vi "Parametric Viewer.vi"(8 "Error In":errorcluster, 11 "F6XX_In":T1) -> (0 "Error Out":errorcluster, 3 "F6XX_Out":T1)   [LabVIEW 2023]
uses:
  type defs/F6_ERD_Control.ctl
panel:
  in  "?":enum32{"F6XX"}(tab)
  in  "Stop":bool
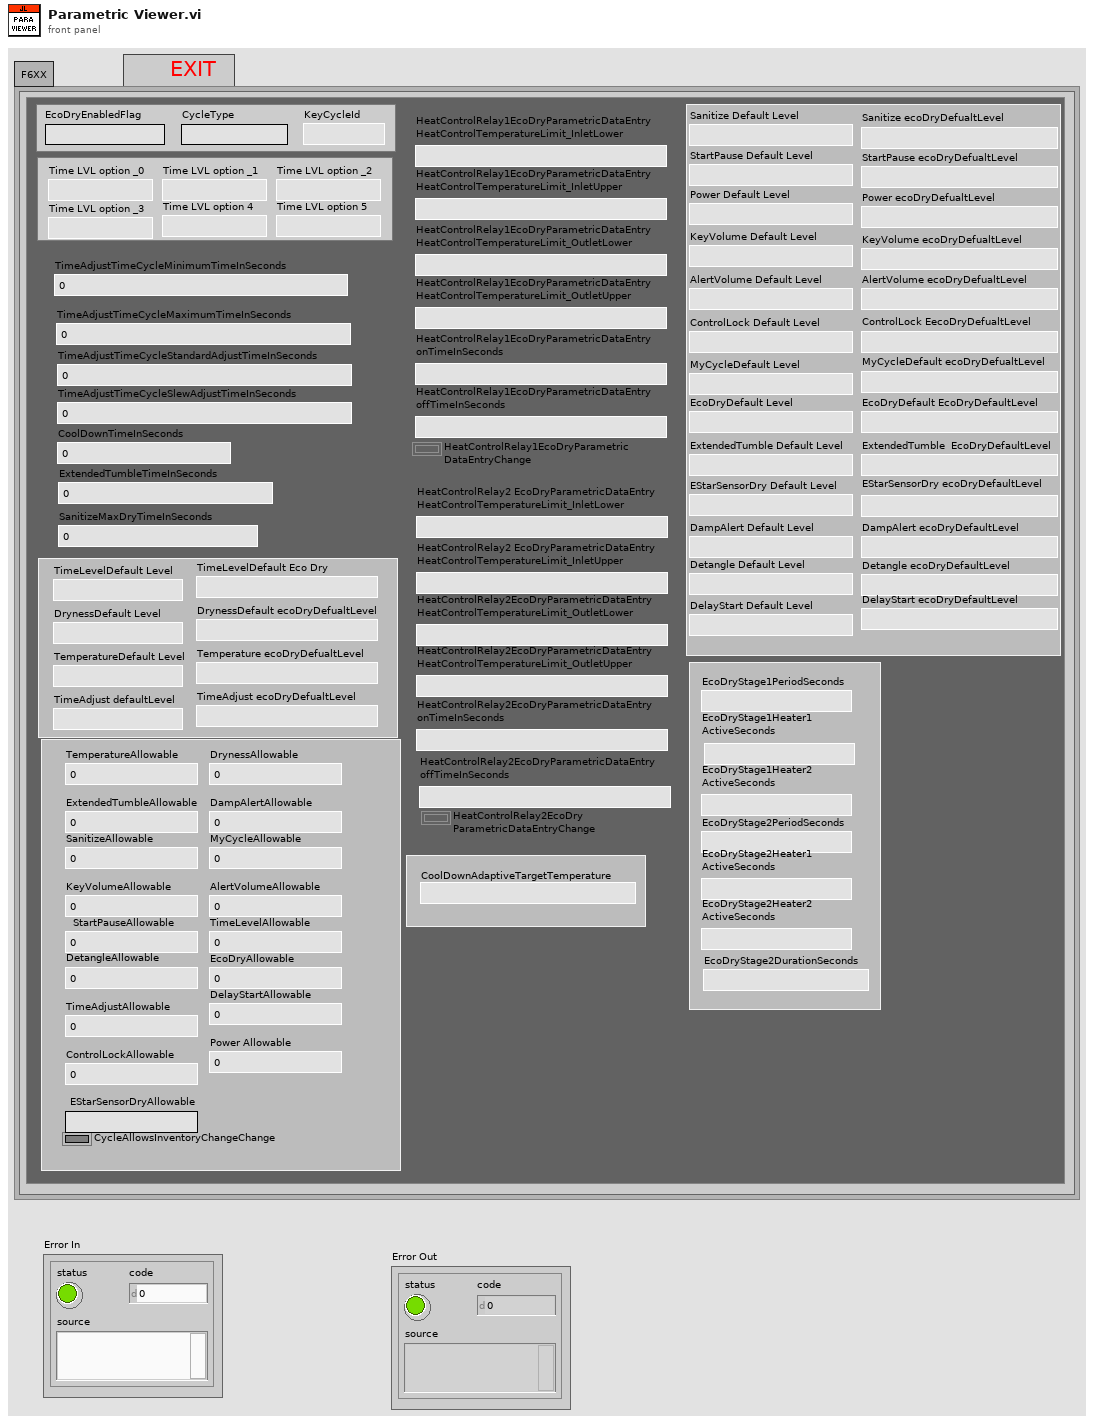
[diagram p1: front panel]
types:
  T1 = typedef "F6_ERD_Control.ctl" = cluster{"EcoDryEnabledFlag":string, "KeyCycleId":u8, "CycleType":string, "Time LVL option 5":u32, "Time LVL option 4":u32, "Time LVL option _3":u32, "Time LVL option _2":u32, "Time LVL option _1":u32, "Time LVL option _0":u32, "CoolDownTimeInSeconds":u32, "TimeAdjustTimeCycleMinimumTimeInSeconds":u32, "TimeAdjustTimeCycleMaximumTimeInSeconds":u32, "TimeAdjustTimeCycleStandardAdjustTimeInSeconds":u32, "TimeAdjustTimeCycleSlewAdjustTimeInSeconds":u32, "ExtendedTumbleTimeInSeconds":u32, "SanitizeMaxDryTimeInSeconds":u32, "TemperatureDefault Level":u8, "Temperature ecoDryDefualtLevel":u8, "DrynessDefault Level":u8, "DrynessDefault ecoDryDefualtLevel":u8, "TimeAdjust defaultLevel":u8, "TimeAdjust ecoDryDefualtLevel":u8, "TimeLevelDefault Level":u8, "TimeLevelDefault Eco Dry":u8, "EStarSensorDry Default Level":u8, "EStarSensorDry ecoDryDefaultLevel":u8, "EcoDryDefault Level":u8, "EcoDryDefault EcoDryDefaultLevel ":u8, "ExtendedTumble Default Level":u8, "ExtendedTumble  EcoDryDefaultLevel":u8, "Sanitize Default Level":u8, "Sanitize ecoDryDefualtLevel":u8, "MyCycleDefault Level":u8, "MyCycleDefault ecoDryDefualtLevel":u8, "StartPause Default Level":u8, "StartPause ecoDryDefualtLevel":u8, "Power Default Level":u8, "Power ecoDryDefualtLevel":u8, "KeyVolume Default Level":u8, "KeyVolume ecoDryDefualtLevel":u8, "AlertVolume Default Level":u8, "AlertVolume ecoDryDefualtLevel":u8, "ControlLock Default Level":u8, "ControlLock EecoDryDefualtLevel":u8, "HeatControlRelay1EcoDryParametricDataEntry\nHeatControlTemperatureLimit_InletLower":u16, "HeatControlRelay1EcoDryParametricDataEntry\nHeatControlTemperatureLimit_InletUpper":u16, "HeatControlRelay1EcoDryParametricDataEntry\nHeatControlTemperatureLimit_OutletLower":u16, "HeatControlRelay1EcoDryParametricDataEntry\nHeatControlTemperatureLimit_OutletUpper":u16, "HeatControlRelay1EcoDryParametricDataEntry\nonTimeInSeconds":u8, "HeatControlRelay1EcoDryParametricDataEntry\noffTimeInSeconds":u8, "HeatControlRelay1EcoDryParametric\nDataEntryChange ":bool, "HeatControlRelay2 EcoDryParametricDataEntry\nHeatControlTemperatureLimit_InletLower":u16, "HeatControlRelay2 EcoDryParametricDataEntry\nHeatControlTemperatureLimit_InletUpper ":u16, "HeatControlRelay2EcoDryParametricDataEntry\nHeatControlTemperatureLimit_OutletLower ":u16, "HeatControlRelay2EcoDryParametricDataEntry\nHeatControlTemperatureLimit_OutletUpper":u16, "HeatControlRelay2EcoDryParametricDataEntry\nonTimeInSeconds ":u8, "HeatControlRelay2EcoDryParametricDataEntry\noffTimeInSeconds ":u8, "HeatControlRelay2EcoDry\nParametricDataEntryChange":bool, "DampAlert Default Level":u8, "DampAlert ecoDryDefaultLevel":u8, "Detangle Default Level ":u8, "Detangle ecoDryDefaultLevel":u8, "DelayStart Default Level":u8, "DelayStart ecoDryDefaultLevel":u8, "CycleAllowsInventoryChangeChange":bool, "TemperatureAllowable":u8, "DrynessAllowable":u8, "TimeLevelAllowable":u8, "EcoDryAllowable":u8, "ExtendedTumbleAllowable":u8, "DampAlertAllowable":u8, "DetangleAllowable":u8, "DelayStartAllowable":u8, "SanitizeAllowable":u8, "MyCycleAllowable":u8, "TimeAdjustAllowable":u8, "Power Allowable":u8, "KeyVolumeAllowable":u8, "AlertVolumeAllowable":u8, "ControlLockAllowable":u8, "EStarSensorDryAllowable":string, "StartPauseAllowable":u8, "EcoDryStage1Heater2\nActiveSeconds":u32, "EcoDryStage2PeriodSeconds":u32, "EcoDryStage2Heater1\nActiveSeconds":u32, "EcoDryStage2Heater2\nActiveSeconds":u32, "EcoDryStage1Heater1\nActiveSeconds":u32, "EcoDryStage1PeriodSeconds":u32, "EcoDryStage2DurationSeconds":u32, "CoolDownAdaptiveTargetTemperature":u16}
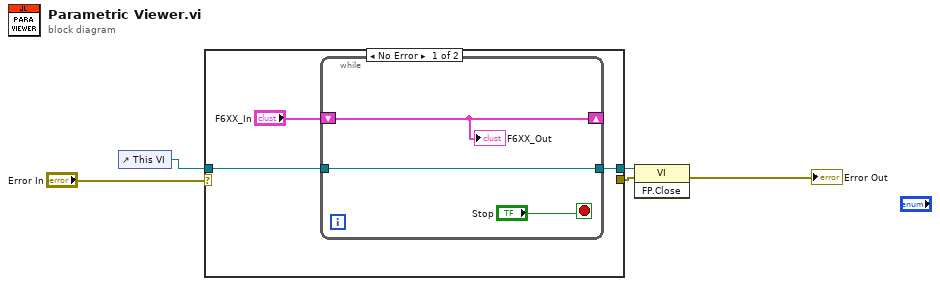
[diagram p0: block diagram]
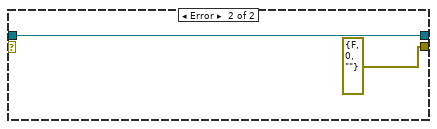
[diagram p2: hidden frame]
diagram:
  n1 = control-ref of="This VI"() -> (w4:refnum<vi>)
  n2 = case shown="No Error" "Error In" {
    tunnel: [w8 w13] -> w5
    tunnel: w4 -> [w6 w13]
    tunnel: [_ errorcluster {"status"=FALSE, "code"=0, "source"=""} ("error IO")] -> w1
    frame No Error {
      n3 = while {
        tunnel: [w9] -> w8
        shift-right: [w10] -> _
        shift-left: "F6XX_In" -> [w10]
        tunnel: w6 -> [w9]
        stop <- "Stop" stop-if-true
        "F6XX_Out" <- w10
      }
    }
    frame Error {
    }
  }
  n4 = invoke class="VI" method="FP.Close"(reference=w5, error in=w1) -> (error out=→"Error Out":errorcluster)  [unwired: 1 in, 2 out]
